vi "SignalRecovery7280Lock-inAmp.vi"() -> ()   [LabVIEW 2021]
panel:
  in  "Tab Control":T1(tab)
  in  "Serial Port Setting":T2={"stop bits "=10, "flow control (0:none)"=0, "parity (none)"=enum."None", "data bits (8)"=8, "termination char (LF)"=10, "baud rate"=19200, "resource name"="COM7", "timeout (ms)"=10000} {"baud rate" items=["110"=110, "300"=300, "600"=600, "1200"=1200, "2400"=2400, "4800"=4800, "9600"=9600, "19200"=19200, "38400"=38400, "57600"=57600, "115200"=115200, "230400"=230400, "460800"=460800, "921600"=921600, "1000000"=1000000, "2000000"=2000000, "4000000"=4000000]; "termination char (LF)" format="%02x"; "data bits (8)" min=5 max=8 step=1; "flow control (0:none)" items=["None", "XON/XOFF", "RTS/CTS", "XON/XOFF & RTS/CTS", "DTR/DSR", "XON/XOFF & DTR/DSR"]; "stop bits" items=["1.0"=10, "1.5"=15, "2.0"=20]}
  out "Y":dbl format="%#_6p"
  out "X":dbl format="%#_6p"
  out "Frequency":dbl=1.0 min=0.0 max=360.0 step=0.001 format="%#.3p"
  in  "Auto Phase":bool
  in  "Cluster":T3={"Voltage Input Mode"=0, "Input Shield Mode"=0, "Sensitivity"=0, "AC Gain"=0, "Automatic"=0, "Line Filter"=0, "Reference"=0, "Reference Source"=0, "Ref. Harmonic"=1, "Ref. Phase (degree)"=1.0, "Output Filter Slope"=0, "Time Constant"=0, "Synchronous Filter"=0, "Output Expansion"=0, "Output CH1"=0, "Output CH2"=0, "Oscillator Amp (Vrms)"=1.0, "Oscillator Freq (Hz)"=1.0} {"Oscillator Freq (Hz)" min=0.0 max=2000000.0 format="%#_6p"; "Oscillator Amp (Vrms)" min=0.0 max=1.0 step=0.001 format="%#.3f"; "Output CH2" items=["X % (2.5 V FS)", "Y % (2.5 V FS)", "R % (2.5 V FS)", "Phase (30 deg/V, 0V=0deg)", "Phase (30 deg/V, -9V=0deg)", "Noise % (2.5 V FS)", "Raitio (10 x X%/ADC 1)", "Ratio log10(10 x X%/ADC1)", "Equation 1", "Equation 2", "X2 % (2.5 V FS)", "Y2 % (2.5 V FS)", "R2 % (2.5 V FS)", "Phase2 (30 deg/V, 0V=0deg)", "Phase2 (30 deg/V, -9V=0deg)"]; "Output CH1" items=["X % (2.5 V FS)", "Y % (2.5 V FS)", "R % (2.5 V FS)", "Phase (30 deg/V, 0V=0deg)", "Phase (30 deg/V, -9V=0deg)", "Noise % (2.5 V FS)", "Raitio (10 x X%/ADC 1)", "Ratio log10(10 x X%/ADC1)", "Equation 1", "Equation 2", "X2 % (2.5 V FS)", "Y2 % (2.5 V FS)", "R2 % (2.5 V FS)", "Phase2 (30 deg/V, 0V=0deg)", "Phase2 (30 deg/V, -9V=0deg)"]; "Output Expansion" items=["Off", "Expand X", "Expand Y", "Expand X & Y"]; "Synchronous Filter" items=["Disabled", "Enabled"]; "Time Constant" items=["500 us"=8, "1 ms"=9, "2 ms"=10, "5 ms"=11, "10 ms"=12, "20 ms"=13, "50 ms"=14, "100 ms"=15, "200 ms"=16, "500 ms"=17, "1 s"=18, "2 s"=19, "5 s"=20, "10 s"=21, "20 s"=22, "50 s"=23, "100 s"=24, "200 s"=25, "500 s"=26, "1 ks"=27, "2 ks"=28, "5 ks"=29, "10 ks"=30, "20 ks"=31, "50 ks"=32, "100 ks"=33, ""=34]; "Output Filter Slope" items=["6 dB/oct", "12 dB/oct", "18 dB/oct (TC>=0.5ms)", "24 dB/oct (TC>=0.5ms)"]; "Ref. Phase (degree)" min=0.0 max=360.0 step=0.001 format="%#.3f"; "Ref. Harmonic" min=1 max=32 step=1; "Reference Source" items=["Internal", "Ext. Logic", "Ext. Analog"]; "Reference" items=["Single / Virtual", "Dual Harmonic", "Dual Reference"]; "Line Filter" items=["Off", "50 Hz", "100 Hz", "50 Hz & 100 Hz"]; "Automatic" items=["No", "Yes"]; "AC Gain" items=["0 dB", "6 dB", "14 dB", "20 dB", "26 dB", "34 dB", "40 dB", "46 dB", "54 dB", "60 dB", "66 dB"]; "Sensitivity" items=["10 nV"=3, "20 nV"=4, "50 nV"=5, "100 nV"=6, "200 nV"=7, "500 nV"=8, "1 uV"=9, "2 uV"=10, "5 uV"=11, "10 uV"=12, "20 uV"=13, "50 uV"=14, "100 uV"=15, "200 uV"=16, "500 uV"=17, "1 mV"=18, "2 mV"=19, "5 mV"=20, "10 mV"=21, "20 mV"=22, "50 mV"=23, "100 mV"=24, "200 mV"=25, "500 mV"=26, "1 V"=27]; "Input Shield Mode" items=["Ground", "Float (1kOhm to GND)"]; "Voltage Input Mode" items=["Both inputs grounded", "A input only", "-B input only", "A-B differential"]}
  out "Serial Port":refnum<visa-resource-name>
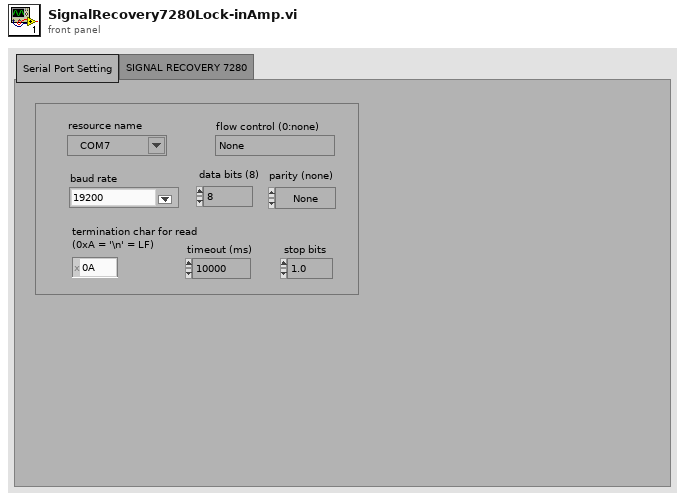
[diagram p1: front panel]
types:
  T1 = enum32{"Serial Port Setting", "SIGNAL RECOVERY 7280"}
  T2 = cluster{"stop bits ":u16, "flow control (0:none)":u16, "parity (none)":enum16{"None", "Odd", "Even", "Mark", "Space"}, "data bits (8)":u16, "termination char (LF)":u8, "baud rate":u32, "resource name":refnum<visa-resource-name>, "timeout (ms)":u32}
  T3 = cluster{"Voltage Input Mode":u16, "Input Shield Mode":u16, "Sensitivity":u16, "AC Gain":u16, "Automatic":u16, "Line Filter":u16, "Reference":u16, "Reference Source":u16, "Ref. Harmonic":u32, "Ref. Phase (degree)":dbl, "Output Filter Slope":u16, "Time Constant":u16, "Synchronous Filter":u16, "Output Expansion":u16, "Output CH1":u16, "Output CH2":u16, "Oscillator Amp (Vrms)":dbl, "Oscillator Freq (Hz)":dbl}
  T4 = cluster{"Operation":enum16{"read", "write"}, "Data":string, "Queue":refnum<queue>}
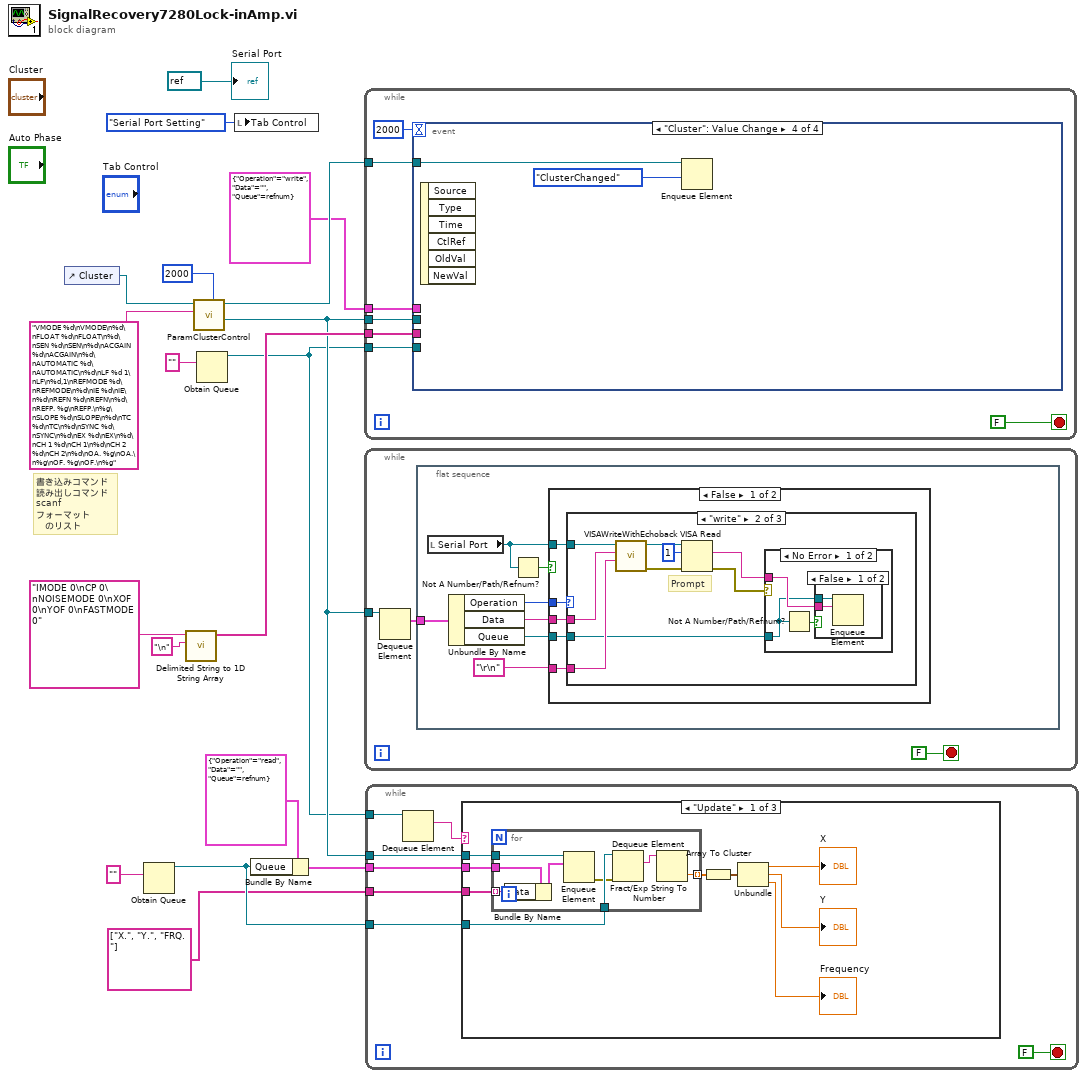
[diagram p0: block diagram]
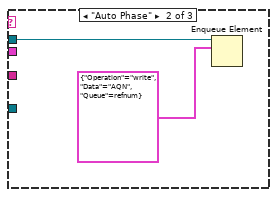
[diagram p2: hidden frame]
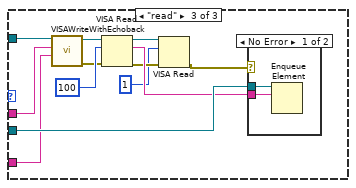
[diagram p7: hidden frame]
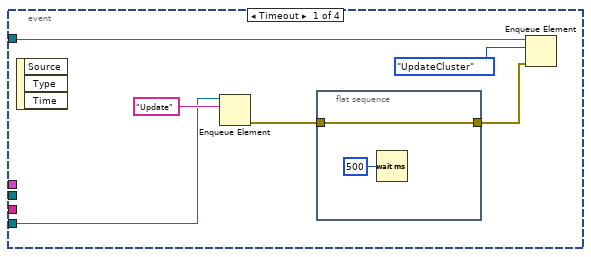
[diagram p10: hidden frame]
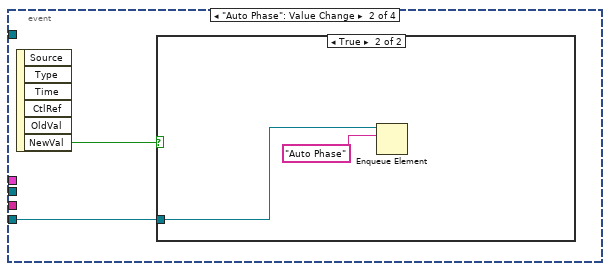
[diagram p11: hidden frame]
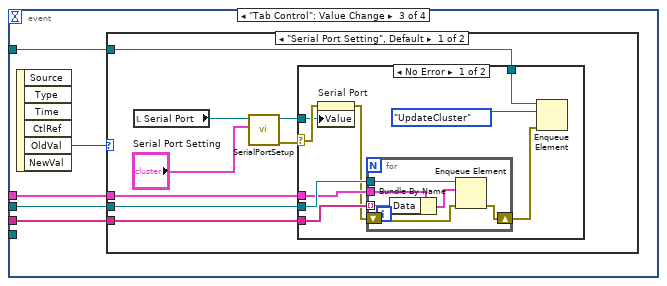
[diagram p13: hidden frame]
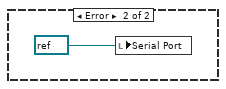
[diagram p14: hidden frame]
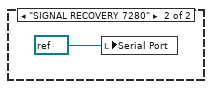
[diagram p15: hidden frame]
diagram:
  # "書き込みコマンド\n読み出しコマンド\nscanf フォーマット\n　のリスト"
  n1 = control-ref of="Cluster"() -> (w18:refnum<vi>)
  n2 = Obtain Queue(element data type="" ("String")) -> (queue out=w4:refnum<queue>)  [unwired: 4 in, 2 out]
  n3 = call <vilib>:"Delimited String to 1D String Array.vi"("delimiter"="\n", "delimited string"="IMODE 0\nCP 0\nNOISEMODE 0\nXOF 0\nYOF 0\nFASTMODE 0") -> ("string array"=w10:string[])  [unwired: 9 in]
  n4 = call "ParamClusterControl.vi"("timeout in ms (100ms)"=2000, "SetGetCommands"="VMODE %d\nVMODE\n%d\nFLOAT %d\nFLOAT\n%d\nSEN %d\nSEN\n%d\nACGAIN %d\nACGAIN\n%d\nAUTOMATIC %d\nAUTOMATIC\n%d\nLF %d 1\nLF\n%d,1\nREFMODE %d\nREFMODE\n%d\nIE %d\nIE\n%d\nREFN %d\nREFN\n%d\nREFP. %g\nREFP.\n%g\nSLOPE %d\nSLOPE\n%d\nTC %d\nTC\n%d\nSYNC %d\nSYNC\n%d\nEX %d\nEX\n%d\nCH 1 %d\nCH 1\n%d\nCH 2 %d\nCH 2\n%d\nOA. %g\nOA.\n%g\nOF. %g\nOF.\n%g", "Cluster ref"=w18) -> ("IO queue out"=w6:refnum<queue>, "Command queue"=w15:refnum<queue>)  [unwired: 7 in]
  n5 = Obtain Queue(element data type="" ("String")) -> (queue out=w1:refnum<queue>)  [unwired: 4 in, 2 out]
  n6 = local write "Tab Control"(T1."Serial Port Setting" ("Tab Control")) -> ()
  n7 = Bundle By Name(cluster=T4 {"Operation"=enum."read", "Data"="", "Queue"=refnum} ("element"), "Queue"=w4) -> (w5:T4)
  n8 = while {
    tunnel: w15 -> [w24]
    tunnel: w6 -> [w22]
    tunnel: T4 {"Operation"=enum."write", "Data"="", "Queue"=refnum} ("element") -> [w21]
    tunnel: w10 -> [w20]
    tunnel: w1 -> [w19]
    stop <- FALSE stop-if-true
    n9 = event shown="[3] \"Cluster\": Value Change" {
      selector: _ -> [_ _ _ _]
      dyn-events: _ -> [_ _ _ _]
      timeout: 2000 -> [_ _ _ _]
      tunnel: w24 -> [w31 _ w41 w69]
      tunnel: w22 -> [_ _ w40 _]
      tunnel: w21 -> [_ _ w39 _]
      tunnel: w20 -> [_ _ w38 _]
      tunnel: w19 -> [w27 w34 _ _]
      event Timeout {
        n10 = event-data() -> ()  [unwired: 1 in, 3 out]
        n11 = Enqueue Element(queue=w27, element="Update") -> (error out=w28:errorcluster)  [unwired: 2 in, 2 out]
        n12 = flat-sequence {
          tunnel: w28 -> [w32]
          tunnel: [w32] -> w26
          frame #0 {
            n13 = Wait (ms)(milliseconds to wait=u32 500) -> ()  [unwired: 1 out]
          }
        }
        n14 = Enqueue Element(queue=w31, element=enum16{"UpdateCluster", "ClusterChanged"}."UpdateCluster", error in (no error)=w26) -> ()  [unwired: 1 in, 3 out]
      }
      event "Auto Phase": Value Change {
        n15 = event-data() -> ("NewVal"=w35:bool)  [unwired: 1 in, 5 out]
        n16 = case shown="True" w35 {
          tunnel: w34 -> [_ w37]
          frame False {
          }
          frame True {
            n17 = Enqueue Element(queue=w37, element="Auto Phase") -> ()  [unwired: 2 in, 3 out]
          }
        }
      }
      event "Tab Control": Value Change {
        n18 = event-data() -> ("OldVal"=w42:T1)  [unwired: 1 in, 5 out]
        n19 = case shown="\"Serial Port Setting\", Default" w42 {
          tunnel: w41 -> [w43 _]
          tunnel: w40 -> [w46 _]
          tunnel: w39 -> [w45 _]
          tunnel: w38 -> [w44 _]
          frame "Serial Port Setting", Default {
            n20 = local read "Serial Port"() -> (w50:refnum<visa-resource-name>)
            n21 = call "SerialPortSetup.vi"("Serial Port Setting"="Serial Port Setting", "VISA resource name (will be closed)"=w50) -> ("error out"=w48:errorcluster, "VISA resource name out"=w47:refnum<visa-resource-name>)  [unwired: 8 in]
            n22 = case shown="No Error" w48 {
              selector: w48 -> [w56 _]
              tunnel: w47 -> [w55 _]
              tunnel: w46 -> [w59 _]
              tunnel: w45 -> [w58 _]
              tunnel: w44 -> [w57 _]
              tunnel: w43 -> [w54 _]
              frame No Error {
                n23 = property on="Serial Port" class="VISAName"(error in=w56, "Value"=w55) -> (error out=w52:errorcluster)  [unwired: 1 in, 1 out]
                n24 = for {
                  tunnel: w59 -> [w65]
                  tunnel: w58 -> [w64]
                  tunnel: w57 -> [w62] mode=indexing
                  shift-right: [w60] -> w51
                  shift-left: w52 -> [w61]
                  n25 = Bundle By Name(cluster=w64, "Data"=w62) -> (w63:T4)
                  n26 = Enqueue Element(queue=w65, element=w63, error in (no error)=w61) -> (error out=w60:errorcluster)  [unwired: 1 in, 2 out]
                }
                n27 = Enqueue Element(queue=w54, element=enum16{"UpdateCluster", "ClusterChanged"}."UpdateCluster", error in (no error)=w51) -> ()  [unwired: 1 in, 3 out]
              }
              frame Error {
                n28 = local write "Serial Port"(refnum<visa-resource-name> refnum ("t")) -> ()
              }
            }
          }
          frame "SIGNAL RECOVERY 7280" {
            n29 = local write "Serial Port"(refnum<visa-resource-name> refnum ("t")) -> ()
          }
        }
      }
      event "Cluster": Value Change {
        n30 = event-data() -> ()  [unwired: 1 in, 6 out]
        n31 = Enqueue Element(queue=w69, element=enum16{"UpdateCluster", "ClusterChanged"}."ClusterChanged") -> ()  [unwired: 2 in, 3 out]
      }
    }
  }
  n32 = while {
    tunnel: w6 -> [w71]
    stop <- FALSE stop-if-true
    n33 = Dequeue Element(queue=w71) -> (element=w70:T4)  [unwired: 2 in, 3 out]
    n34 = flat-sequence {
      tunnel: w70 -> [w78]
      frame #0 {
        n35 = local read "Serial Port"() -> (w76:refnum<visa-resource-name>)
        n36 = Unbundle By Name(w78) -> ("Operation"=w77:enum16{"read", "write"}, "Data"=w74:string, "Queue"=w75:refnum<queue>)
        n37 = Not A Number/Path/Refnum?(number/path/refnum=w76) -> (NaN/Path/Refnum?=w79:bool)
        n38 = case shown="False" w79 {
          tunnel: w77 -> [w84 _]
          tunnel: w76 -> [w83 _]
          tunnel: w74 -> [w82 _]
          tunnel: w75 -> [w81 _]
          tunnel: "\r\n" -> [w80 _]
          frame False {
            n39 = case shown="\"write\"" w84 {
              tunnel: w83 -> [_ w93 w107]
              tunnel: w82 -> [_ w92 w106]
              tunnel: w81 -> [_ w86 w109]
              tunnel: w80 -> [_ w91 w105]
              frame Default {
              }
              frame "write" {
                # "Prompt"
                n40 = call "VISAWriteWithEchoback.vi"("termination"=w91, "write data"=w92, "VISA resource name"=w93) -> ("error out"=w85:errorcluster, "VISA resource name out"=w90:refnum<visa-resource-name>)  [unwired: 6 in, 1 out]
                n41 = VISA Read(VISA resource name=w90, byte count=u32 1, error in (no error)=w85) -> (read buffer=w87:string, error out=w88:errorcluster)  [unwired: 2 out]
                n42 = case shown="No Error" w88 {
                  tunnel: w87 -> [w96 _]
                  tunnel: w86 -> [w95 _]
                  frame No Error {
                    n43 = Not A Number/Path/Refnum?(number/path/refnum=w95) -> (NaN/Path/Refnum?=w94:bool)
                    n44 = case shown="False" w94 {
                      tunnel: w96 -> [w98 _]
                      tunnel: w95 -> [w97 _]
                      frame False {
                        n45 = Enqueue Element(queue=w97, element=w98) -> ()  [unwired: 2 in, 3 out]
                      }
                      frame True {
                      }
                    }
                  }
                  frame Error {
                  }
                }
              }
              frame "read" {
                n46 = call "VISAWriteWithEchoback.vi"("termination"=w105, "write data"=w106, "VISA resource name"=w107) -> ("error out"=w103:errorcluster, "VISA resource name out"=w104:refnum<visa-resource-name>)  [unwired: 6 in, 1 out]
                n47 = VISA Read(VISA resource name=w104, byte count=u32 100, error in (no error)=w103) -> (VISA resource name out=w102:refnum<visa-resource-name>, read buffer=w108:string, error out=w101:errorcluster)  [unwired: 1 out]
                n48 = VISA Read(VISA resource name=w102, byte count=u32 1, error in (no error)=w101) -> (error out=w99:errorcluster)  [unwired: 3 out]
                n49 = case shown="No Error" w99 {
                  tunnel: w109 -> [w112 _]
                  tunnel: w108 -> [w111 _]
                  frame No Error {
                    n50 = Enqueue Element(queue=w112, element=w111) -> ()  [unwired: 2 in, 3 out]
                  }
                  frame Error {
                  }
                }
              }
            }
          }
          frame True {
          }
        }
      }
    }
  }
  n51 = while {
    tunnel: w6 -> [w119]
    tunnel: w5 -> [w118]
    tunnel: w4 -> [w117]
    tunnel: string[] ["X.", "Y.", "FRQ."] -> [w116]
    tunnel: w1 -> [w115]
    stop <- FALSE stop-if-true
    n52 = Dequeue Element(queue=w115) -> (element=w113:string)  [unwired: 2 in, 3 out]
    n53 = case shown="\"Update\"" w113 {
      tunnel: w119 -> [w128 w138 _]
      tunnel: w118 -> [w127 _ _]
      tunnel: w117 -> [w126 _ _]
      tunnel: w116 -> [w125 _ _]
      frame "Update" {
        n54 = for {
          tunnel: w128 -> [w136]
          tunnel: w127 -> [w135]
          tunnel: w126 -> [w133]
          tunnel: w125 -> [w131] mode=indexing
          tunnel: [w129] -> w124 mode=indexing
          n55 = Bundle By Name(cluster=w135, "Data"=w131) -> (w134:T4)
          n56 = Enqueue Element(queue=w136, element=w134) -> (error out=w132:errorcluster)  [unwired: 2 in, 2 out]
          n57 = Dequeue Element(queue=w133, error in (no error)=w132) -> (element=w130:string)  [unwired: 1 in, 3 out]
          n58 = Fract/Exp String To Number(string=w130) -> (number=w129:dbl)  [unwired: 3 in, 1 out]
        }
        n59 = Array To Cluster(array=w124) -> (cluster=w123:cluster{"[0]":dbl, "[1]":dbl, "[2]":dbl})
        n60 = Unbundle(w123) -> ("[0]"=→"X":dbl, "[1]"=→"Y":dbl, "[2]"=→"Frequency":dbl)
      }
      frame "Auto Phase" {
        n61 = Enqueue Element(queue=w138, element=T4 {"Operation"=enum."write", "Data"="AQN", "Queue"=refnum}) -> ()  [unwired: 2 in, 3 out]
      }
      frame Default {
      }
    }
  }
  "Serial Port" <- refnum<visa-resource-name> refnum ("t")
